vi "Bitget 8-bits test.vi"(0 "x":i32) -> (20 "a":dbl, 21 "b":dbl, 22 "c":dbl, 23 "d":dbl, 24 "e":dbl, 25 "f":dbl, 26 "g":dbl, 27 "h":dbl)   [LabVIEW 2020]
uses:
  <vilib>/imath/engines/lvmath2/RunTimeEngine/BuiltInFunctions/bitget/NIMS_bitget(SorS,SorS).vi
  <vilib>/imathl/engines/lvmath/Functions/Error Handling/Create Error.vi
  <vilib>/imath/engines/lvmath2/RunTimeEngine/NodeEndStatement/NIMS_NodeEndStatement_Output.vi
  <instcachedir>/0/NIMS_NodeEndStatement_Output_53EC0D466D134D7ABD903AC30B43404B.lvgen/NIMS_NodeEndStatement_Output_53EC0D466D134D7ABD903AC30B43404B_001.vi
  <vilib>/imath/engines/lvmath2/RunTimeEngine/ErrorHandling/NIMS_Finalize Error.vi
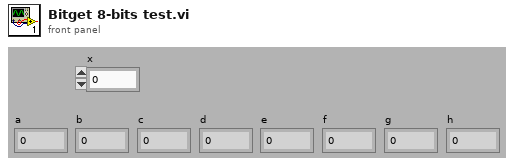
[diagram p1: front panel]
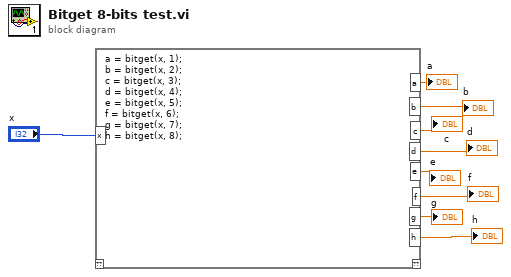
[diagram p0: block diagram]
diagram:
  n1 = mathscript code="a = bitget(x, 1);\nb = bitget(x, 2);\nc = bitget(x, 3);\nd = bitget(x, 4);\ne = bitget(x, 5);\nf = bitget(x, 6);\ng = bitget(x, 7);\nh = bitget(x, 8);"("x"="x") -> ("a"=→"a":dbl, "b"=→"b":dbl, "c"=→"c":dbl, "d"=→"d":dbl, "e"=→"e":dbl, "g"=→"g":dbl, "h"=→"h":dbl, "f"=→"f":dbl)  [unwired: 1 in, 1 out]
